vi "FPGA.vi"() -> ()   [LabVIEW 2020]
uses:
  <vilib>/rvi/DataTransferAndStorage/Container/XNode/niFpgaContainer.xnode
  <vilib>/rvi/interface/RandomDataEmulation/nirviRandomDataFpgaReadWriteTemplate.vi
  <vilib>/rvi/FIFO/Fifo_Resource/nirvififoEmulationWrite.vi
panel:
  out "Sorted array":u8[](array[numeric])
  out "Output Valid":bool
  in  "Input Valid":bool
  in  "Input Array":u8[](array[numeric])=[0, 0, 0, 0, 0, 0, 0, 0]
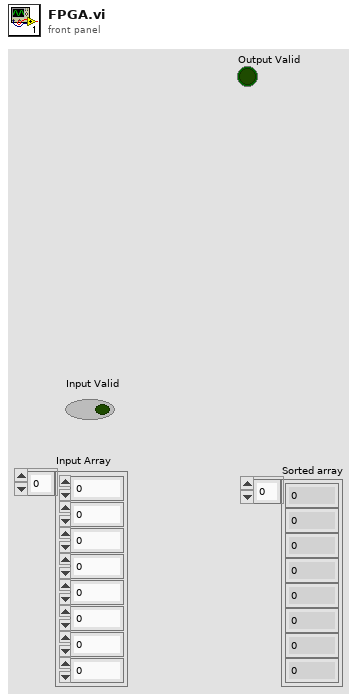
[diagram p1: front panel]
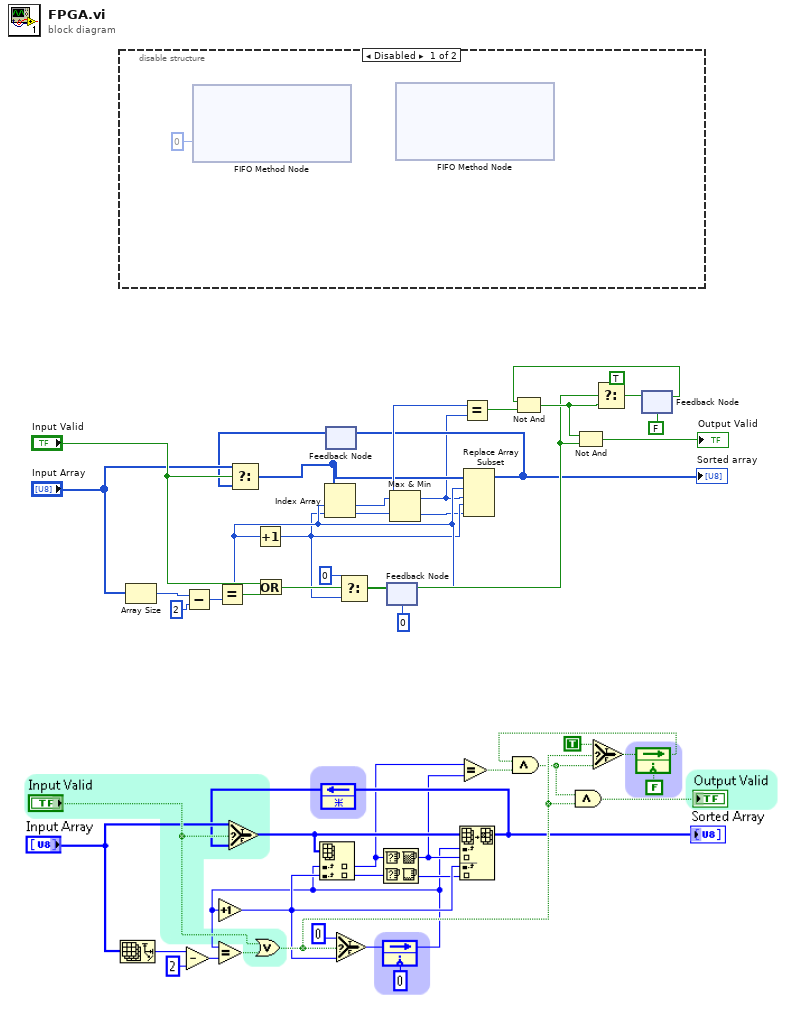
[diagram p0: block diagram]
diagram:
  n1 = disable-structure shown="Disabled" {
    frame Disabled {
      n2 = xnode ("FIFO Method Node")("Timeout"=0) -> ()  [unwired: 1 in, 3 out]
      n3 = xnode ("FIFO Method Node")() -> ()  [unwired: 3 in, 2 out]
    }
    frame Enabled {
    }
  }
  n4 = Array Size(array="Input Array") -> (size(s)=w25:i32)
  n5 = Subtract(x=w25, y=2) -> (x-y=w23:i32)
  n6 = feedback #1() -> (w12:u8[])  [unwired: 1 in]
  n7 = Select(t="Input Array", s="Input Valid", f=w12) -> (s? t:f=w6:u8[])
  n8 = feedback #2(0 ("y")) -> (w4:i32)
  n9 = Equal?(x=w4, y=w23) -> (x = y?=w7:bool)
  n10 = Increment(x=w4) -> (x+1=w2:i32)
  n11 = Or(x="Input Valid", y=w7) -> (x .or. y?=w10:bool)
  n12 = Index Array(array=w6, index #1=w4, index #2=w2) -> (element #1=w20:u8, element #2=w21:u8)
  n13 = Select(t=0 ("y"), s=w10, f=w2) -> (s? t:f=w8:i32)
  n14 = feedback-in #2(w8) -> ()
  n15 = Max & Min(x=w20, y=w21) -> (max(x,y)=w3:u8, min(x,y)=w1:u8)
  n16 = Equal?(x=w20, y=w3) -> (x = y?=w19:bool)
  n17 = Replace Array Subset(array=w6, new element #1=w3, index #1=w4, new element #2=w1, index #2=w2) -> (w5:u8[])
  "Sorted array" <- w5
  n18 = feedback-in #1(w5) -> ()
  n19 = feedback #3(FALSE ("t")) -> (w16:bool)
  n20 = Not And(1:w19, 2:w16) -> (0:w14:bool)
  n21 = Not And(1:w10, 2:w14) -> (0:→"Output Valid":bool)
  n22 = Select(t=TRUE, s=w10, f=w14) -> (s? t:f=w17:bool)
  n23 = feedback-in #3(w17) -> ()
